vi "Fan Temperature Acquisition.vi"(6 "Control Index":i32, 8 "error in (no error)":errorcluster, 9 "channel":T1, 10 "Stream in":refnum<class "Stream.lvclass">, 11 "DAQmx Task In":refnum<k21>) -> (0 "error out":errorcluster, 3 "DAQmx Task Out":refnum<k21>)   [LabVIEW 2020]
uses:
  <extravilib>/ChannelInstances/Tag-bool/))Channel.ctl
  submodules/nominal-streaming-labview-ffi/lv_src/Stream/Stream.lvclass
  <vilib>/DAQmx/read.llb/DAQmx Read (Analog DBL 1Chan 1Samp).vi
  <extravilib>/ChannelInstances/Tag-bool/Read With Abort.vi
  <extravilib>/ChannelInstances/Tag-bool/EndpointRead.vi
  <vilib>/DAQmx/miscellaneous.llb/DAQmx Fill In Error Info.vi
  <extravilib>/ChannelInstances/Tag-bool.lvlib
  submodules/nominal-streaming-labview-ffi/lv_src/Channel/Channel.lvclass
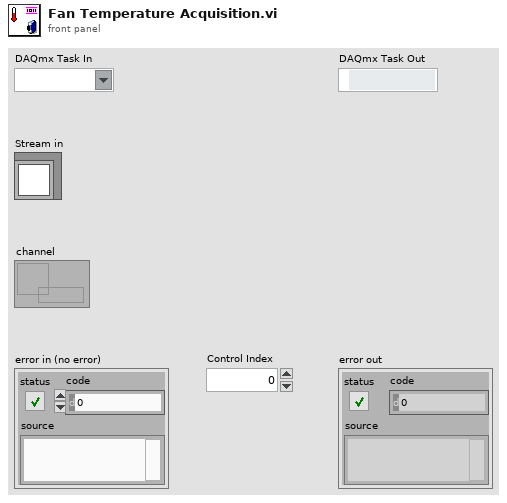
[diagram p1: front panel]
types:
  T1 = typedef "Tag-bool.lvlib/))Channel.ctl" = refnum<queue>
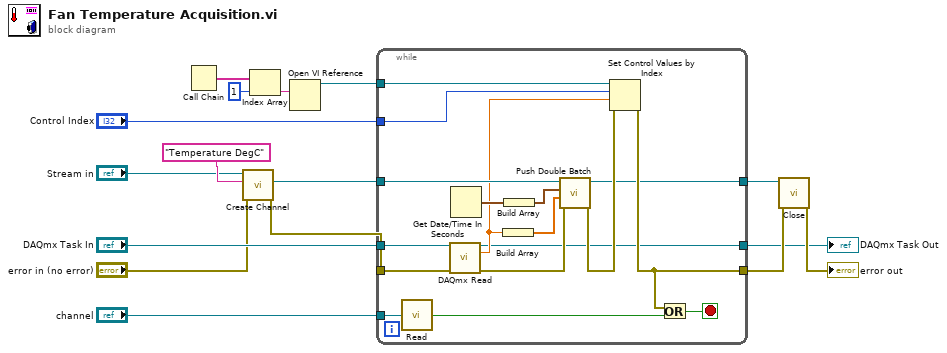
[diagram p0: block diagram]
diagram:
  n1 = Call Chain() -> (call chain=w10:string[])
  n2 = call "Create Channel.vi"("error in (no error)"="error in (no error)", "Channel Name"="Temperature DegC", "Nominal Streaming in"="Stream in") -> ("error out"=w6:errorcluster, "Channel"=w9:refnum<class "Channel.lvclass">)  [unwired: 6 in, 1 out]
  n3 = Index Array(array=w10, index=1) -> (element=w12:string)
  n4 = Open VI Reference(vi path=w12) -> (vi reference=w8:refnum<vi>)  [unwired: 5 in, 1 out]
  n5 = while {
    tunnel: "DAQmx Task In" -> [w33]
    tunnel: w6 -> [w32]
    tunnel: [w19] -> w4
    tunnel: [w18] -> w2
    tunnel: "channel" -> [w30]
    tunnel: w9 -> [w25]
    tunnel: w8 -> [w23]
    tunnel: "Control Index" -> [w21]
    tunnel: [w17] -> w5
    stop <- w31 stop-if-true
    n6 = call <extravilib>:"Read.vi"("channel"=w30) -> ("element"=w29:bool)  [unwired: 1 in, 1 out]
    n7 = call-poly <vilib>:"DAQmx Read.vi"("task/channels in"=w33, "error in"=w32) -> ("task out"=w18:refnum<k21>, "data"=w22:dbl, "error out"=w24:errorcluster)  [unwired: 11 in]
    n8 = Get Date/Time In Seconds() -> (seconds since 1Jan1904=w28:timestamp)
    n9 = Build Array(w22) -> (w27:dbl[])
    n10 = Build Array(w28) -> (w26:timestamp[])
    n11 = call "Push Double Batch.vi"("error in (no error)"=w24, "Values"=w27, "Timestamps"=w26, "Channel in"=w25) -> ("error out"=w20:errorcluster, "Channel out"=w17:refnum<class "Channel.lvclass">)  [unwired: 6 in]
    n12 = Set Control Values by Index(0:w23, 1:w21, 2:w22, 3:w20) -> (11:w19:errorcluster)
    n13 = Or(x=w19, y=w29) -> (x .or. y?=w31:bool)
  }
  "DAQmx Task Out" <- w2
  n14 = call "Close.vi"("error in (no error)"=w4, "Channel in"=w5) -> ("error out"=→"error out":errorcluster)  [unwired: 9 in]
